vi "Transmitter_RSMA - With Timer 16QAM.vi"() -> ()   [LabVIEW 2022 SP3]
uses:
  <instrlib>/niUSRP/niUSRP Write Tx Data (CDB).vi
panel:
  in  "Iterations":i32=10000
  out "Time(s)":sgl format="%#_4g"
  in  "Alpha":dbl(slide)=0.17500000000000002 step=0.005 scale=0.0..1.0
  in  "Tab Control":enum32{"USRP Parameters", "Transmission"}(tab)
  in  "USRP ControledParameters 2":T1={"Active Antenna"="TX1", "Gain (dB)"=0.0, "Carrier Frequency"=2400000000.0, "IQ Rate"=2000000.0, "Active Channel"="0"} {"IQ Rate" format="%#_6p"; "Carrier Frequency" format="%#_6p"; "Gain (dB)" format="%#_6f"}
  in  "Device selection":refnum<k15>="RIO0"
  in  "stop":bool
  out "Error out":errorcluster
  in  "Modulation parameter":T2
  out "Bits length":i32
  out "Bits length 2":i32
  out "Frame Duration":dbl format="%#_6p"
  out "Coerced Parameters":T3={"IQ Rate"=100000.0, "Carrier  Freq."=100000.0, "Gain"=0.0} {"Gain" format="%#_6f"; "Carrier  Freq." format="%#_6p"; "IQ Rate" format="%#_6p"}
  out "Transmitted Waveform":dbl[](graph)
  in  "Message 2":string="ptua. At vero eos et accusam et justo duo dolores et ea rebum. Stet clita kasd gubergren, no sea takimata sanctus est Lorem ipsum dolor sit amet. Lore"
  in  "Message 1":string="Lorem ipsum dolor sit amet, consetetur sadipscing elitr, sed diam nonumy eirmod tempor invidunt ut labore et dolore magna aliquyam erat, sed diam volu"
  in  "error in (no error)":errorcluster
  # "RSMA Transmitter"
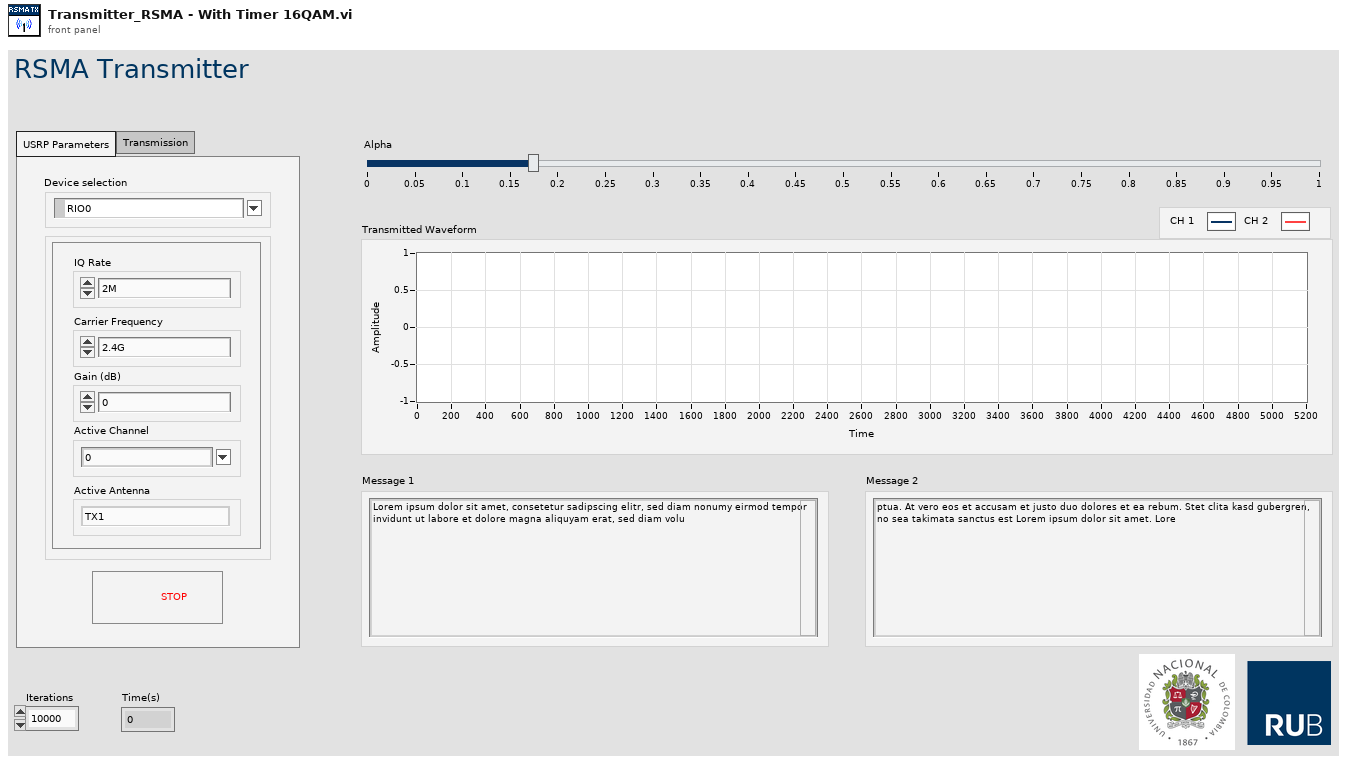
[diagram p1: front panel]
types:
  T1 = cluster{"Active Antenna":string, "Gain (dB)":dbl, "Carrier Frequency":dbl, "IQ Rate":dbl, "Active Channel":string}
  T2 = cluster{"Modulation type":enum16{"QPSK(4QAM)", "64QAM", "16QAM", "BPSK"}, "BCC rate (k/n)":enum16{"1/2", "2/3", "3/4"}}
  T3 = cluster{"IQ Rate":dbl, "Carrier  Freq.":dbl, "Gain":dbl}
  T4 = cluster{"coerced IQ rate":dbl, "coerced carrier frequency":dbl, "coerced gain":dbl}
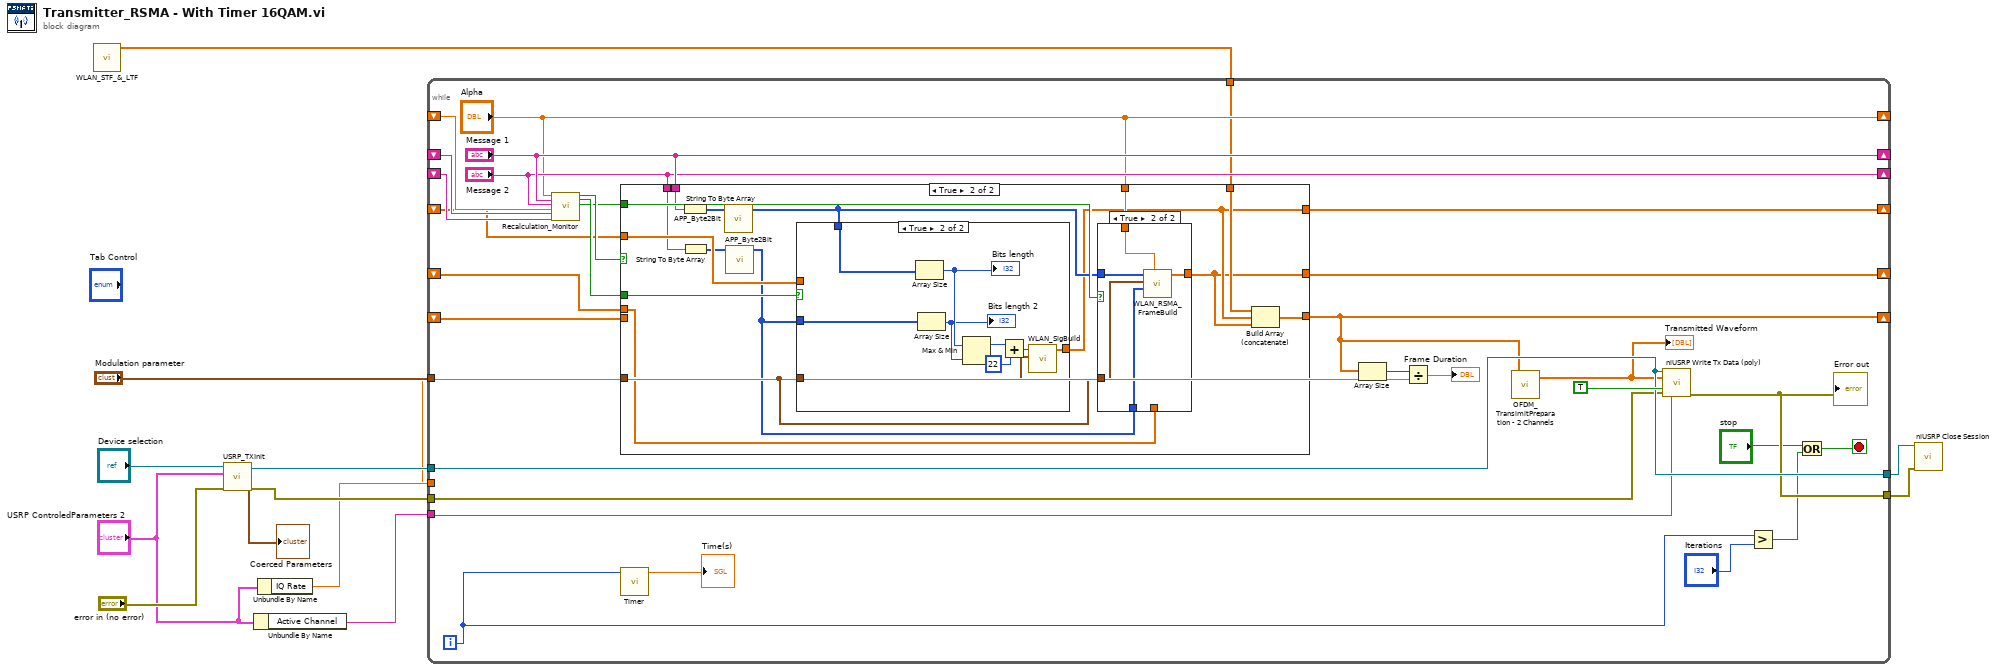
[diagram p0: block diagram]
diagram:
  n1 = call "WLAN_STF_&_LTF.vi"() -> ("STF & LTF"=w1:cdb[])  [unwired: 11 in]
  n2 = call "USRP_TXInit.vi"("device names"="Device selection", "USRP ControledParameters"="USRP ControledParameters 2", "error in (no error)"="error in (no error)") -> ("session handle out"=w11:refnum<k15>, "USRP CoercedParamters"=→"Coerced Parameters":T4, "error out"=w10:errorcluster)  [unwired: 5 in]
  n3 = Unbundle By Name("USRP ControledParameters 2") -> ("Active Channel"=w3:string)
  n4 = Unbundle By Name("USRP ControledParameters 2") -> ("IQ Rate"=w9:dbl)
  n5 = while {
    tunnel: w11 -> [w41]
    tunnel: w10 -> [w21]
    tunnel: w9 -> [w40]
    tunnel: [w41] -> w8
    tunnel: [w39] -> w7
    tunnel: w3 -> [w38]
    shift-right: ["Alpha"] -> _
    shift-left: _ -> [w37]
    shift-right: ["Message 1"] -> _
    shift-left: _ -> [w36]
    shift-right: ["Message 2"] -> _
    shift-left: _ -> [w35]
    tunnel: "Modulation parameter" -> [w29]
    shift-right: [w28] -> _
    shift-left: _ -> [w27]
    shift-right: [w25] -> _
    shift-left: _ -> [w24]
    tunnel: w1 -> [w23]
    shift-right: [w20] -> _
    shift-left: _ -> [w22]
    i -> [w16]
    stop <- w13 stop-if-true
    n6 = call "Recalculation_Monitor.vi"("Alpha"="Alpha", "Message 1"="Message 1", "Message 2"="Message 2", "Alpha old"=w37, "Message 1 old"=w36, "Message 2 old"=w35) -> ("Recalculate?"=w34:bool, "Recalculate SIG"=w33:bool, "Recalculate OFDM"=w32:bool)  [unwired: 11 in]
    n7 = case shown="True" w34 {
      tunnel: w33 -> [_ w63]
      tunnel: w32 -> [_ w62]
      tunnel: "Message 1" -> [_ w57]
      tunnel: "Message 2" -> [_ w58]
      tunnel: w29 -> [_ w54]
      tunnel: [w47 w50] -> w28
      tunnel: w27 -> [w47 w61]
      tunnel: "Alpha" -> [_ w53]
      tunnel: [w46 w49] -> w25
      tunnel: w24 -> [w46 w52]
      tunnel: w23 -> [_ w51]
      tunnel: [w45 w48] -> w20
      tunnel: w22 -> [w45 _]
      frame False {
      }
      frame True {
        n8 = String To Byte Array(string=w57) -> (unsigned byte array=w59:u8[])
        n9 = String To Byte Array(string=w58) -> (unsigned byte array=w60:u8[])
        n10 = call "APP_Byte2Bit.vi"("input byte stream"=w59) -> ("output bit stream"=w55:i8[])  [unwired: 10 in]
        n11 = call "APP_Byte2Bit.vi"("input byte stream"=w60) -> ("output bit stream"=w56:i8[])  [unwired: 10 in]
        n12 = case shown="True" w63 {
          tunnel: w54 -> [_ w71]
          tunnel: [w70 w77] -> w50
          tunnel: w61 -> [w70 _]
          tunnel: w56 -> [_ w73]
          tunnel: w55 -> [_ w72]
          frame False {
          }
          frame True {
            n13 = Array Size(array=w72) -> (size(s)=w79:i32)
            "Bits length" <- w79
            n14 = Array Size(array=w73) -> (size(s)=w78:i32)
            "Bits length 2" <- w78
            n15 = Max & Min(x=w79, y=w78) -> (max(x,y)=w75:i32)  [unwired: 1 out]
            n16 = Add(x=w75, y=22) -> (x+y=w76:i32)
            n17 = call "WLAN_SigBuild.vi"("Data bit length"=w76, "Modulation parameter"=w71) -> ("symbols"=w77:cdb[])  [unwired: 7 in, 1 out]
          }
        }
        n18 = case shown="True" w62 {
          tunnel: w56 -> [_ w69]
          tunnel: w55 -> [_ w68]
          tunnel: w54 -> [_ w67]
          tunnel: w53 -> [_ w66]
          tunnel: [w64 w65] -> w49
          tunnel: w52 -> [w64 _]
          frame False {
          }
          frame True {
            n19 = call "WLAN_RSMA_FrameBuild.vi"("Alpha"=w66, "data in 2"=w69, "Modulation parameter"=w67, "data in"=w68) -> ("output array"=w65:cdb[])  [unwired: 6 in, 1 out]
          }
        }
        n20 = Build Array (concatenate)(w51, w50, w49) -> (w48:cdb[])
      }
    }
    n21 = call "Timer.vi"("index"=w16) -> ("Time(s)"=→"Time(s)":sgl)  [unwired: 10 in]
    n22 = Array Size(array=w20) -> (size(s)=w43:i32)
    n23 = Divide(x=w43, y=w40) -> (x/y=→"Frame Duration":dbl)
    n24 = call "OFDM_TransimitPreparation - 2 Channels.vi"("array"=w20) -> ("output array"=w19:cdb[])  [unwired: 8 in, 2 out]
    "Transmitted Waveform" <- w19
    n25 = call-poly <instrlib>:"niUSRP Write Tx Data (poly).vi"("session handle"=w41, "channel list"=w38, "data"=w19, "end of data?"=TRUE, "error in (no error)"=w21) -> ("error out"=w39:errorcluster)  [unwired: 9 in, 1 out]
    "Error out" <- w39
    n26 = Greater?(x=w16, y="Iterations") -> (0:w14:bool)
    n27 = Or(x="stop", y=w14) -> (x .or. y?=w13:bool)
  }
  n28 = call <instrlib>:"niUSRP Close Session.vi"("session handle"=w8, "error in (no error)"=w7) -> ()  [unwired: 13 in, 1 out]
